vi "MultiplyVI.vi"(8 "B":dbl, 11 "A":dbl) -> (3 "Product":dbl)   [LabVIEW 2023]
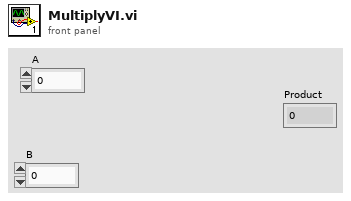
[diagram p1: front panel]
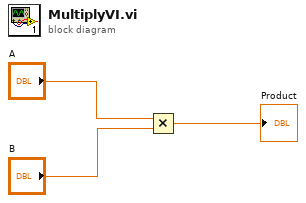
[diagram p0: block diagram]
diagram:
  n1 = Multiply(x="A", y="B") -> (x*y=→"Product":dbl)
